vi "Remove From Parent.vi"(6 "Unique ID":string, 8 "error in (no error)":errorcluster, 10 "Linked List Definition":refnum<class "Linked List Definition.lvclass">, 11 "Linked List in":refnum<class "Linked List.lvclass">) -> (0 "error out":errorcluster, 3 "Linked List out":refnum<class "Linked List.lvclass">)   [LabVIEW 2019, in "Linked Lists.lvlib" / "Linked List.lvclass"]
uses:
  <vilib>/gpm_packages/@cs/linked-list/Source/Linked List/Linked List/Linked List.lvclass
  <vilib>/gpm_packages/@cs/linked-list/Source/Linked List/Linked List Definition/Linked List Definition.lvclass
  <vilib>/gpm_packages/@cs/linked-list/Source/Linked List/Linked List/Linked List.lvclass/Linked List.ctl
  <vilib>/gpm_packages/@cs/lookup-table/Source/LookupTable/LookupTable.lvclass/LookupTable.ctl
  9da57b77-c7cd-4a51-a2ff-b97e5f401819.vi
  d2a87fe5-5aaf-4518-b2c3-133ef3c660e6.vi
  <vilib>/gpm_packages/@cs/lookup-table/Source/LookupTable/Read Table Reference.vi
  9da57b77-c7cd-4a51-a2ff-b97e5f401819.vi/eb9663ae-16ae-49f2-bd36-b832ecb14fee.vi
  d2a87fe5-5aaf-4518-b2c3-133ef3c660e6.vi/9e565620-04bd-443b-8dad-32c81adcbf40.vi
  <vilib>/gpm_packages/@cs/lookup-table/Source/LookupTable/LookupTable.lvclass
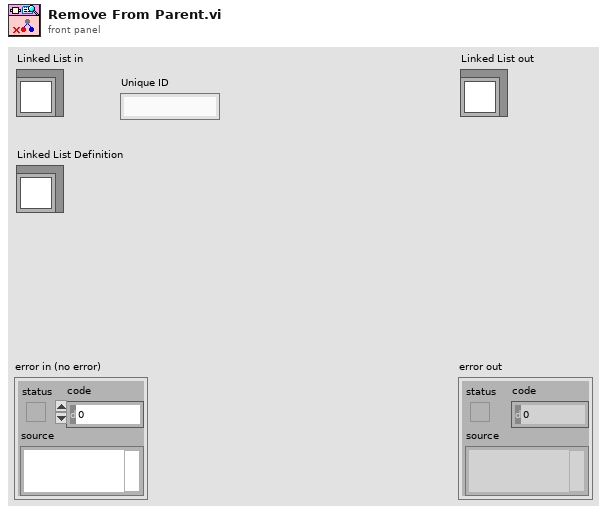
[diagram p1: front panel]
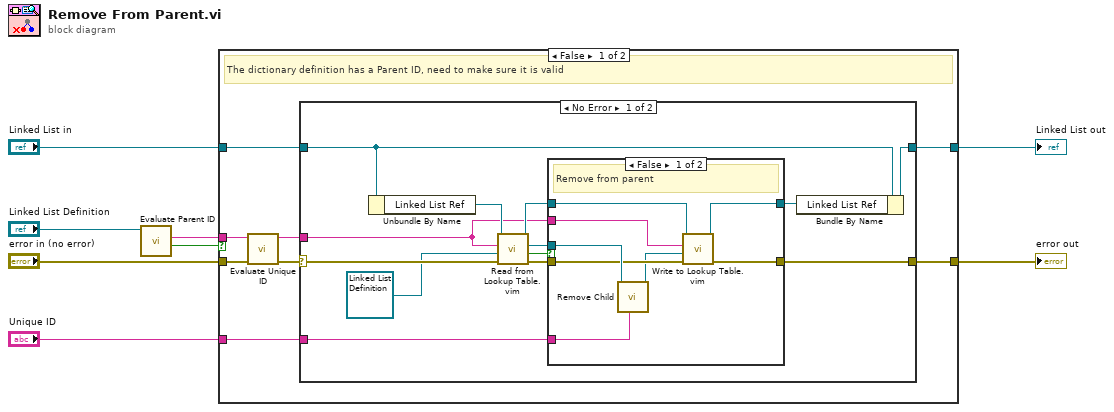
[diagram p0: block diagram]
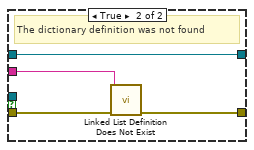
[diagram p2: hidden frame]
diagram:
  n1 = call <vilib>:"Evaluate Parent ID.vi"("Linked List Definition in"="Linked List Definition") -> ("Invalid Parent ID"=w5:bool, "Parent ID"=w4:string)  [unwired: 8 in, 1 out]
  n2 = case shown="False" w5 {
    tunnel: w4 -> [w16 _]
    tunnel: [w10 w45] -> w7
    tunnel: "Linked List in" -> [w14 w45]
    tunnel: "error in (no error)" -> [w15 w44]
    tunnel: [w12 w44] -> w2
    tunnel: "Unique ID" -> [w9 _]
    frame False {
      # "The dictionary definition has a Parent ID, need to make sure it is valid"
      n3 = call <vilib>:"Evaluate Unique ID.vi"("error in (no error)"=w15, "Unique ID"=w16) -> ("error out"=w13:errorcluster, "Unique ID Out"=w11:string)  [unwired: 8 in]
      n4 = case shown="No Error" w13 {
        selector: w13 -> [w28 w42]
        tunnel: w14 -> [w19 w43]
        tunnel: [w22 w42] -> w12
        tunnel: w11 -> [w21 _]
        tunnel: [w18 w43] -> w10
        tunnel: w9 -> [w20 _]
        frame No Error {
          n5 = Unbundle By Name(w19) -> ("Linked List Ref"=w29:refnum<data-value>)
          n6 = call "Read from Lookup Table.vim"("error in (no error)"=w28, "Type"=refnum<class "Linked List Definition.lvclass"> refnum ("Linked List.lvlib:Linked List Definition.lvclass"), "Item Name"=w21, "LookupTable Reference"=w29) -> ("error out"=w23:errorcluster, "Not Found?"=w26:bool, "Value"=w24:refnum<class "Linked List Definition.lvclass">, "LookupTable Reference Out"=w25:refnum<data-value>)  [unwired: 4 in]
          n7 = case shown="False" w26 {
            tunnel: w25 -> [w34 w38]
            tunnel: w24 -> [w37 _]
            tunnel: [w35 w40] -> w22
            tunnel: w23 -> [w36 w41]
            tunnel: w21 -> [w32 w39]
            tunnel: w20 -> [w30 _]
            tunnel: [w31 w38] -> w17
            frame False {
              # "Remove from parent"
              n8 = call <vilib>:"Remove Child.vi"("Unique ID"=w30, "Linked List Definition in"=w37) -> ("Linked List Definition out"=w33:refnum<class "Linked List Definition.lvclass">)  [unwired: 9 in]
              n9 = call "Write to Lookup Table.vim"("error in (no error)"=w36, "Item"=w33, "Item Name"=w32, "LookupTable Reference"=w34) -> ("error out"=w35:errorcluster, "LookupTable Reference Out"=w31:refnum<data-value>)  [unwired: 5 in, 1 out]
            }
            frame True {
              # "The dictionary definition was not found"
              n10 = call <vilib>:"Linked List Definition Does Not Exist.vi"("Error In"=w41, "Unique ID"=w39) -> ("Error Out"=w40:errorcluster)  [unwired: 9 in]
            }
          }
          n11 = Bundle By Name(cluster=w19, "Linked List Ref"=w17) -> (w18:refnum<class "Linked List.lvclass">)
        }
        frame Error {
        }
      }
    }
    frame True {
      # "The dictionary definition does not have a valid parent ID, so it does not need to be removed.  This should not generate an error."
    }
  }
  "error out" <- w2
  "Linked List out" <- w7
